vi "State.vi"(7 "State":T1, 8 "error in (no error)":errorcluster, 10 "Data in":variant, 11 "StateData in":T2) -> (0 "error out":errorcluster, 3 "StateData out":T2)   [LabVIEW 2019, in "Project Properties.lvlib"]
doc: "Handles the <b>State</b> command.\n\nCreated by: Ryan Pacini"
uses:
  Project Properties.lvlib
  State Data.ctl
  VI Property.ctl
  State.ctl
  <vilib>/Utility/miscctls.llb/LVPoint32TypeDef.ctl
  <vilib>/Utility/sysdir.llb/System Directory Type.ctl
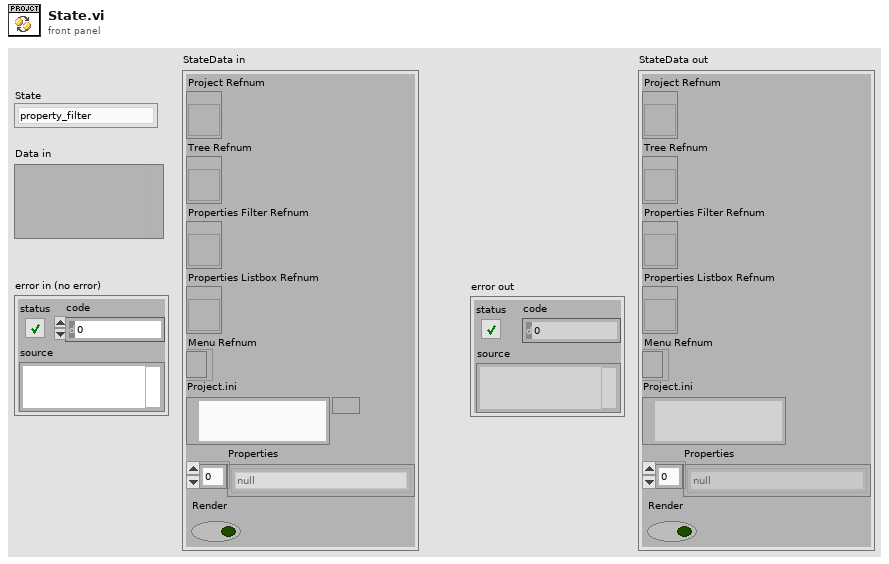
[diagram p1: front panel]
types:
  T1 = typedef "Project Properties.lvlib/State.ctl" = enum8{"property_filter", "property_select", "property_menu_activation", "property_menu_selection", "tree_double_click", "tree_menu_activation", "tree_menu_selection", "export_config"}
  T2 = typedef "Project Properties.lvlib/State Data.ctl" = cluster{"Project Refnum":refnum<vi>, "Tree Refnum":refnum<vi>, "Properties Filter Refnum":refnum<vi>, "Properties Listbox Refnum":refnum<vi>, "Menu Refnum":refnum<k9>, "Project.ini":path, "Properties":T3[], "Render":bool}
  T3 = typedef "Project Properties.lvlib/VI Property.ctl" = enum8{"null", "Auto Logging:Log at Finish", "Auto Logging:Log File Path", "Auto Logging:Print at Finish", "Auto Preallocate Arrays and Strings", "Automatic Error Handling", "BD Master Wizard", "Block Diagram", "Block Diagram Window:Alignment Grid Size", "Block Diagram Window:Native Window", "Block Diagram Window:Open", "Block Diagram Window:Origin", "Block Diagram Window:State", "Block Diagram Window:Window Bounds", "Block Diagram Window:Window Interface", "Callers' Names", "Callers' Paths", "Compiled:Code Complexity", "Compiled:Last Compiled With", "Compiler:Generated Code Profiling Result", "Compiler:Generated Code Profiling Settings", "Connector Pane:Checksum Ignore Dynamic Dispatch v2", "Connector Pane:Checksum v3", "Connector Pane:DataType", "Connector Pane:Reference", "Connector Pane:Set", "Contains Compiled Code", "Context:Has Edits In Another Context", "Context:Has Edits In This Context", "Context:Is Reserved In Other Context", "Context:Is Reserved In This Context", "Control VI Type", "Did Recompile InThis Version", "Do Not Show Save Changes Dialog", "Edit Mode On Open", "Execution highlighting?", "Execution:Allow Debugging", "Execution:Close After Call", "Execution:Compiled With SSE", "Execution:Did Compiler Or User Approve Inlining", "Execution:Inline Enum", "Execution:Inline Is Allowed", "Execution:Inline SubVI", "Execution:Inline SubVI If Possible", "Execution:Is Reentrant", "Execution:Preferred Exec System", "Execution:Priority", "Execution:Reentrancy Type", "Execution:Retain Wire Values", "Execution:Run When Opened", "Execution:Show Front Panel On Call", "Execution:Show Front Panel On Load", "Execution:Shrink Large Buffer Threshold", "Execution:Shrink Large Buffers", "Execution:SSE Runtime Optimization", "Execution:State", "Execution:Suspend On Call", "Expand When Dropped As SubVI", "Front Panel", "Front Panel RefNum TD", "Front Panel Window:Alignment Grid Size", "Front Panel Window:Allow Runtime PopUp", "Front Panel Window:Behavior", "Front Panel Window:Closeable", "Front Panel Window:Custom Title", "Front Panel Window:Highlight Return Button", "Front Panel Window:Is Floating", "Front Panel Window:Is Frontmost", "Front Panel Window:Keep Window Proportions", "Front Panel Window:Minimizable", "Front Panel Window:Minimum Size", "Front Panel Window:Monitor", "Front Panel Window:Native Window", "Front Panel Window:Panel Bounds", "Front Panel Window:Resizable", "Front Panel Window:Run VI Transparently", "Front Panel Window:Show Menu Bar", "Front Panel Window:State", "Front Panel Window:Title", "Front Panel Window:Title Bar Visible", "Front Panel Window:Transparency", "Front Panel Window:Window Bounds", "Front Panel Window:Window Interface", "Has MathScript Nodes", "Help:Document Path", "Help:Document Tag", "Help:Document Web URL", "Help:Examples Exist", "Help:Use Web URL", "Hide Instance VI Caption On Drop", "History:Always Add Comments At Save", "History:Entire Text", "History:Prompt for Comments At Close", "History:Prompt for Comments At Save", "History:Record Application Comments", "History:Revision Number", "History:Use Defaults", "Inline Callees", "Is Clone VI", "Is Generic", "Is In Packed Library", "Is Instance", "Is Probe", "Is Running Interactively", "Is Skinned", "Is System VI", "Is VI Paused?", "Is XNode VI", "Item ID", "Ladder VI Needs Scripting", "Library", "Library:Private", "Library:Version", "Metrics:Advanced", "Metrics:Block Diagram Loaded", "Metrics:Code Size", "Metrics:Front Panel Loaded", "Metrics:Number of clones", "Metrics:Size of Block Diagram", "Metrics:Size of Front Panel", "Metrics:Total Data Size", "Modifications:Block Diagram Mods Bitset", "Modifications:Front Panel Mods Bitset", "Modifications:User Changes", "Modifications:VI Modifications Bitset", "Modifications:VI Signatures", "Modifications:VI User Code GUID", "No Clone If Instance VI", "Number of Non-Proxy Callers", "Overload Info", "Owning Application", "Printing:Block Diagram Scaling?", "Printing:Front Panel Scaling?", "Printing:Header Content:Date Printed?", "Printing:Header Content:Modify Date?", "Printing:Header Content:Page Number?", "Printing:Header Content:VI Icon?", "Printing:Header Content:VI Name?", "Printing:Header Content:VI Path?", "Printing:Margins", "Printing:Page Headers?", "Printing:Page Orientation", "Purgative", "Run-Time Menu Path", "Saved Version", "Statechart:Is Sub Panel Editable", "Statechart:Supress Parse", "Suppress Data Manager", "Suppress Instance VI Halo", "Suppress Transact Info", "Suppress Type Prop", "Tagged And Not Edited", "Terminal Bounds[]", "Tool Bar:Show Abort Button", "Tool Bar:Show Free Run Button", "Tool Bar:Show Run Button", "Tool Bar:Visible", "Tool Kit Attr", "VI Clone Name", "VI Compile Time", "VI Description", "VI Linker Errors", "VI Name", "VI Path", "VI Type"}
  T4 = typedef "LVPoint32TypeDef.ctl" = cluster{"Horizontal":i32, "Vertical":i32}
  T5 = enum16{"open", "replace", "create", "open or create", "replace or create", "replace or create with confirmation"}
  T6 = typedef "System Directory Type.ctl" = i32
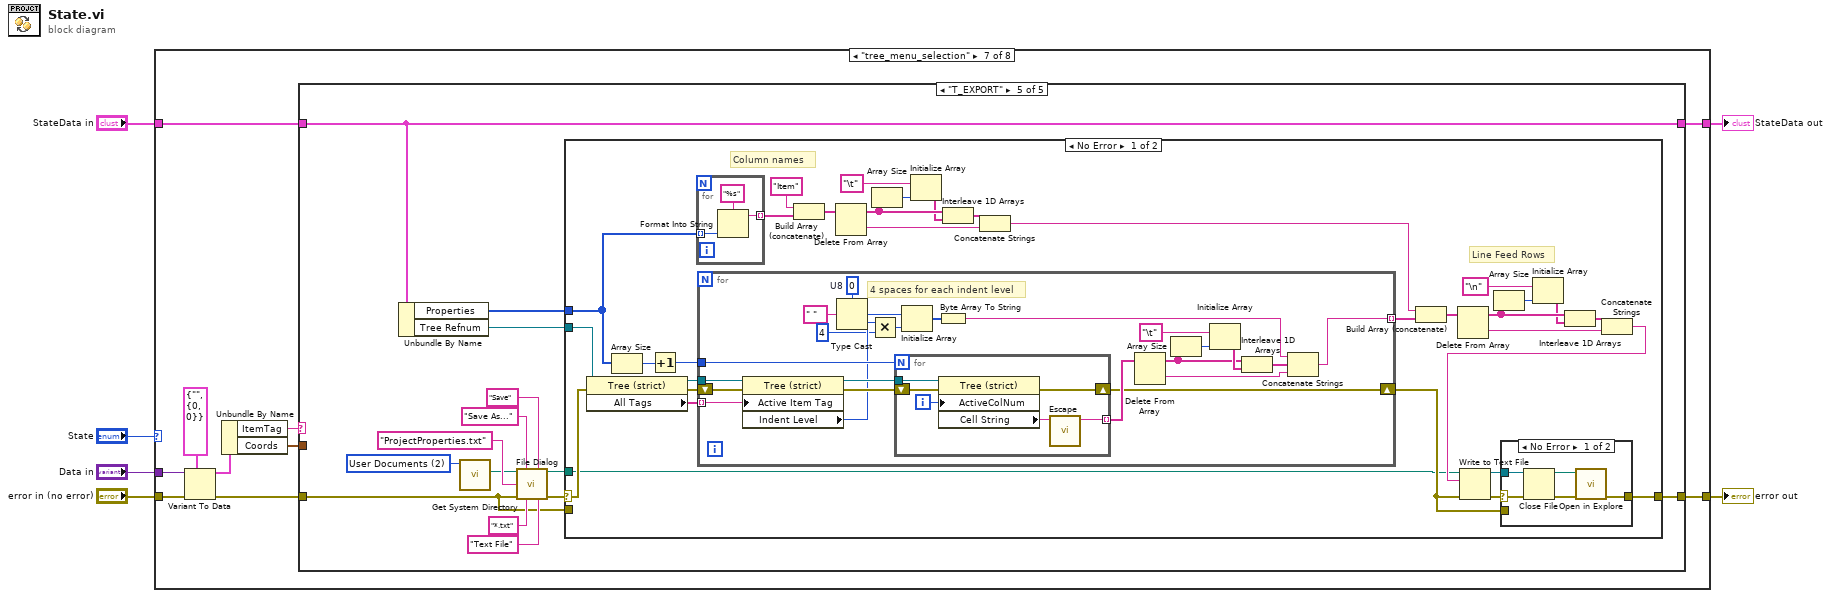
[diagram p0: block diagram]
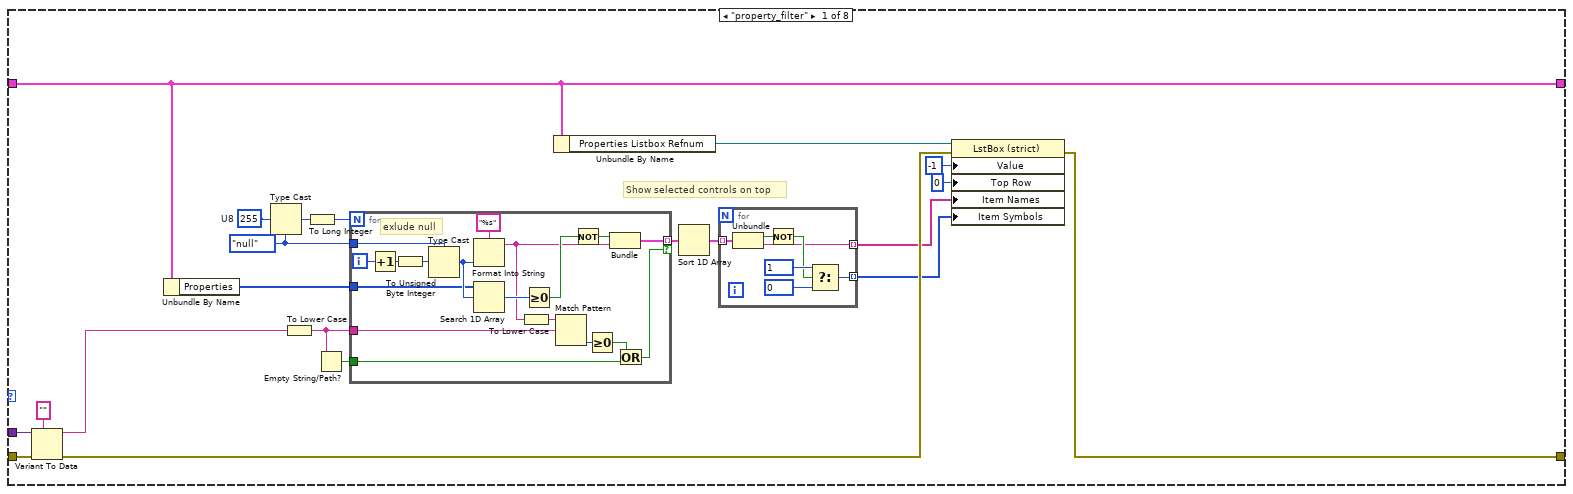
[diagram p2: hidden frame]
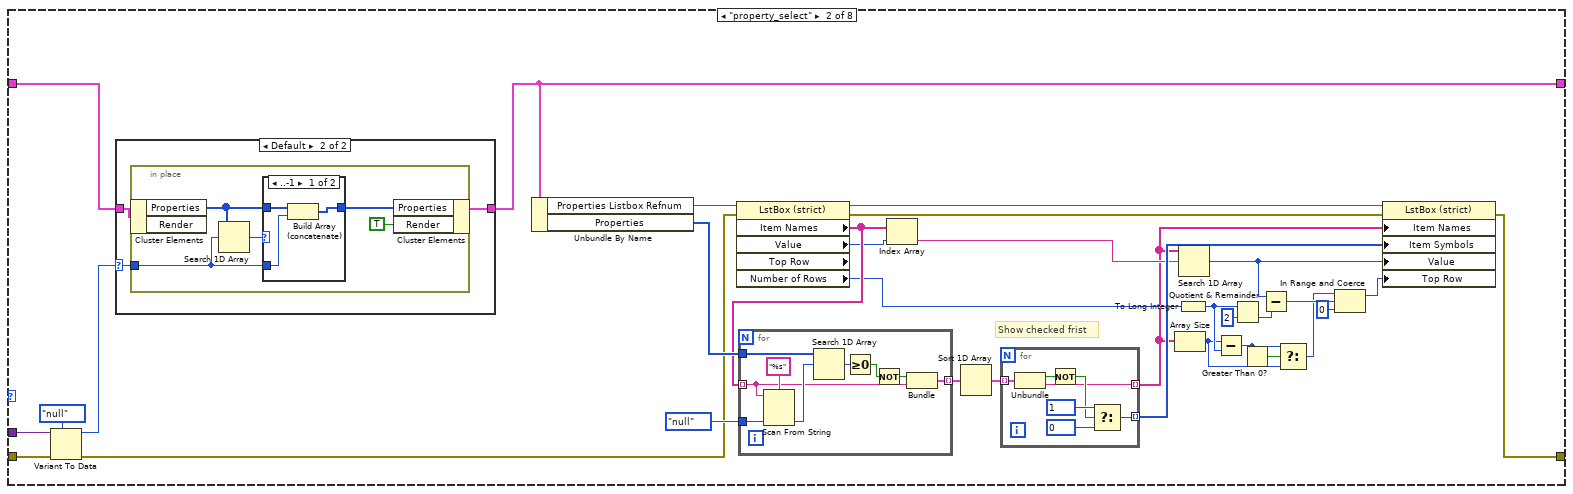
[diagram p3: hidden frame]
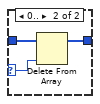
[diagram p5: hidden frame]
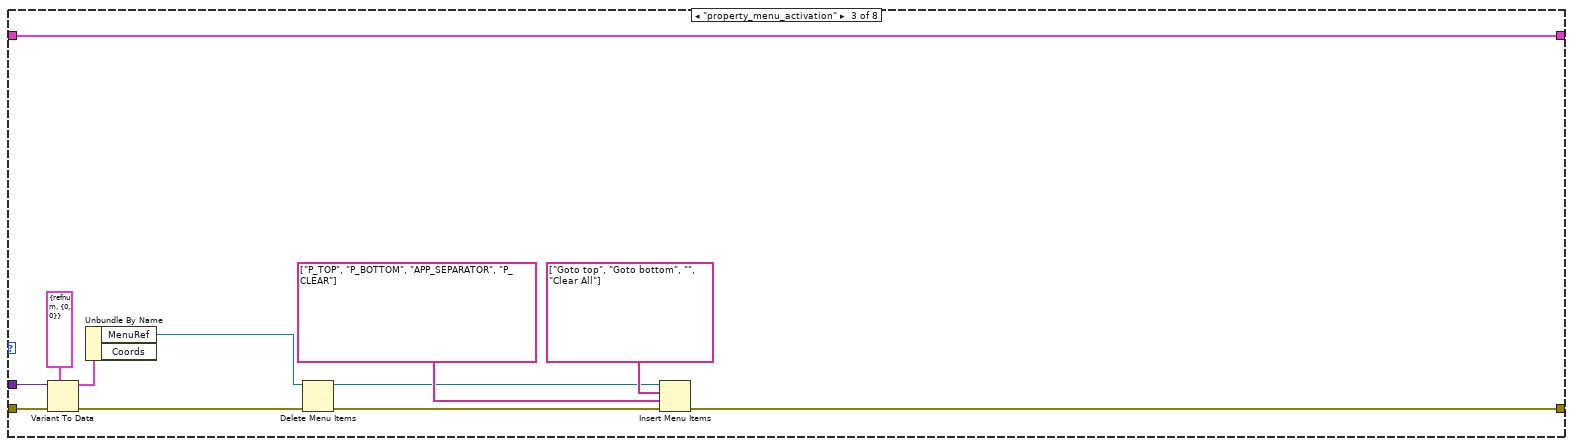
[diagram p6: hidden frame]
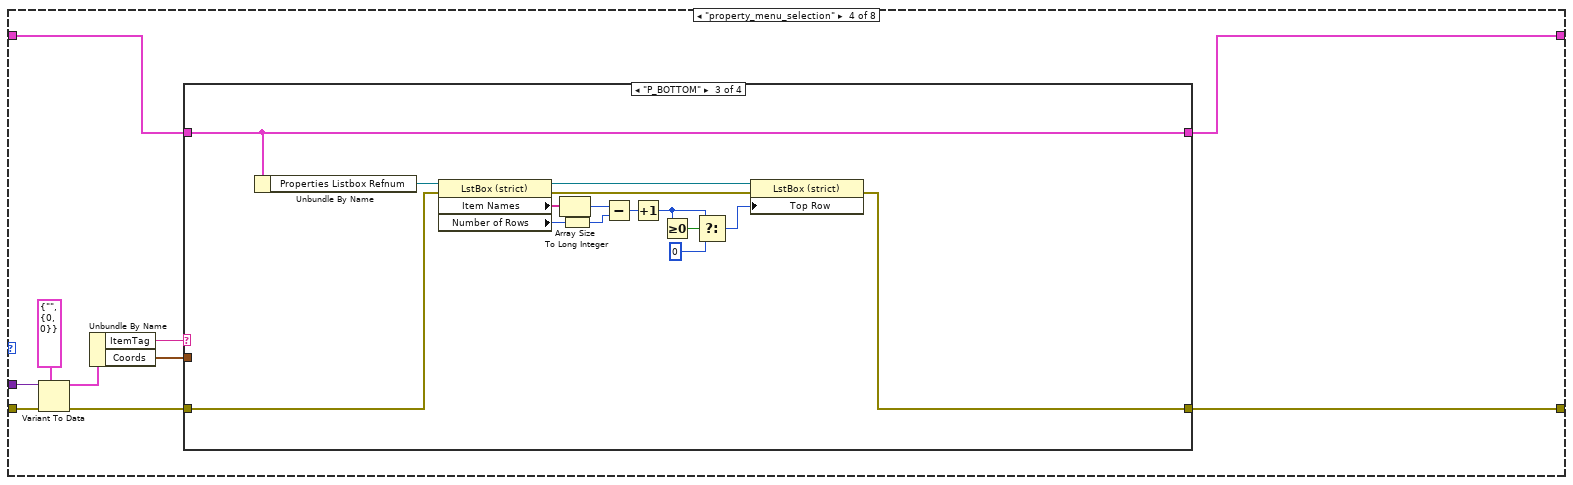
[diagram p7: hidden frame]
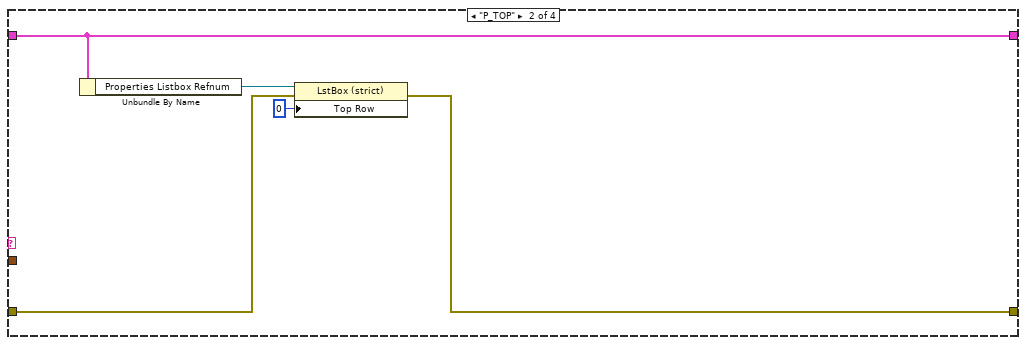
[diagram p9: hidden frame]
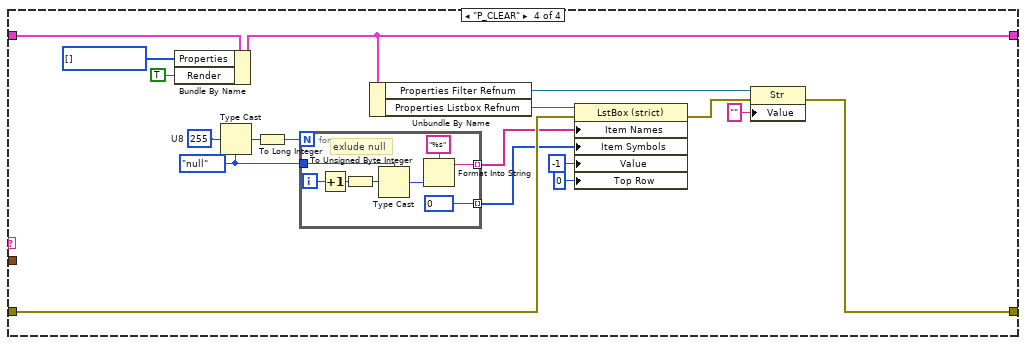
[diagram p10: hidden frame]
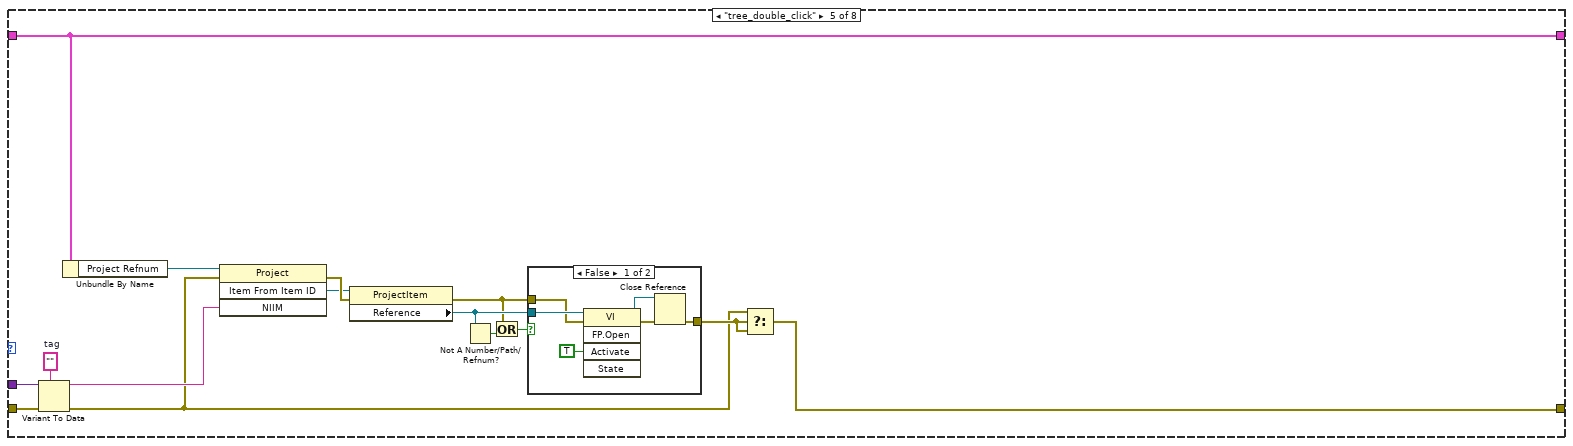
[diagram p11: hidden frame]
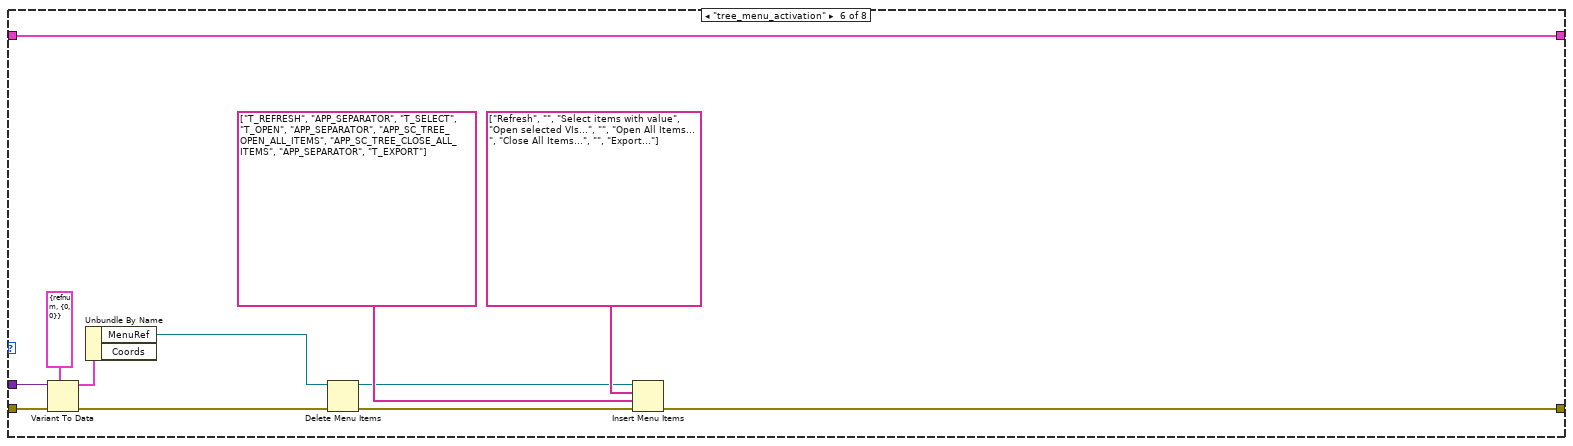
[diagram p13: hidden frame]
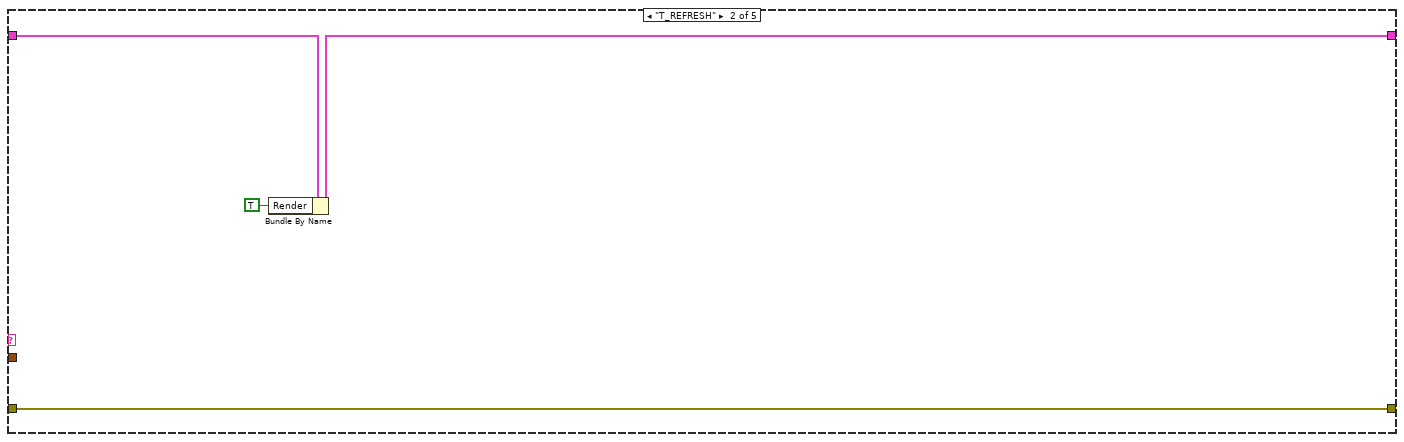
[diagram p15: hidden frame]
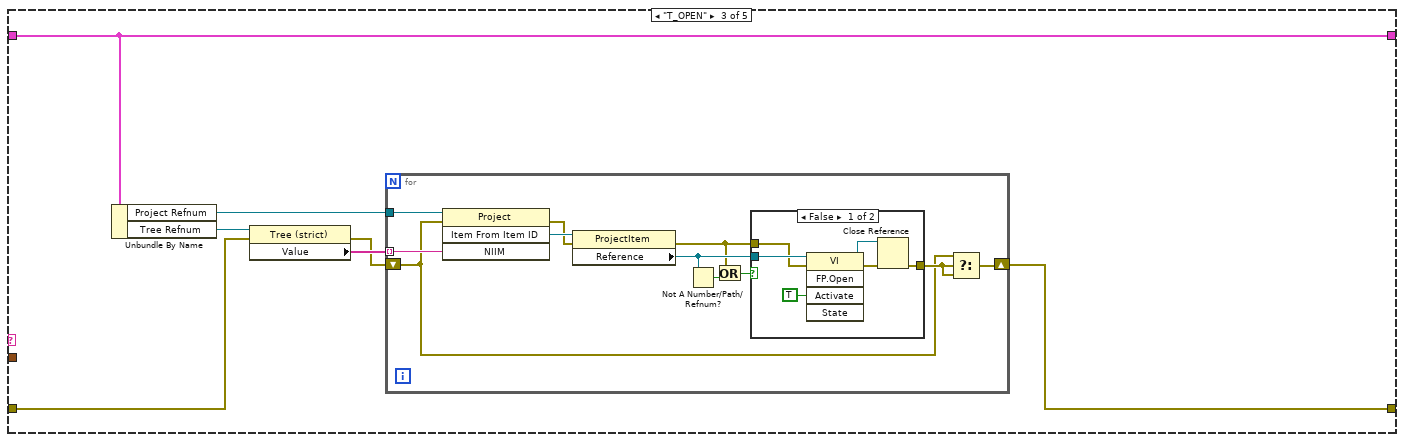
[diagram p16: hidden frame]
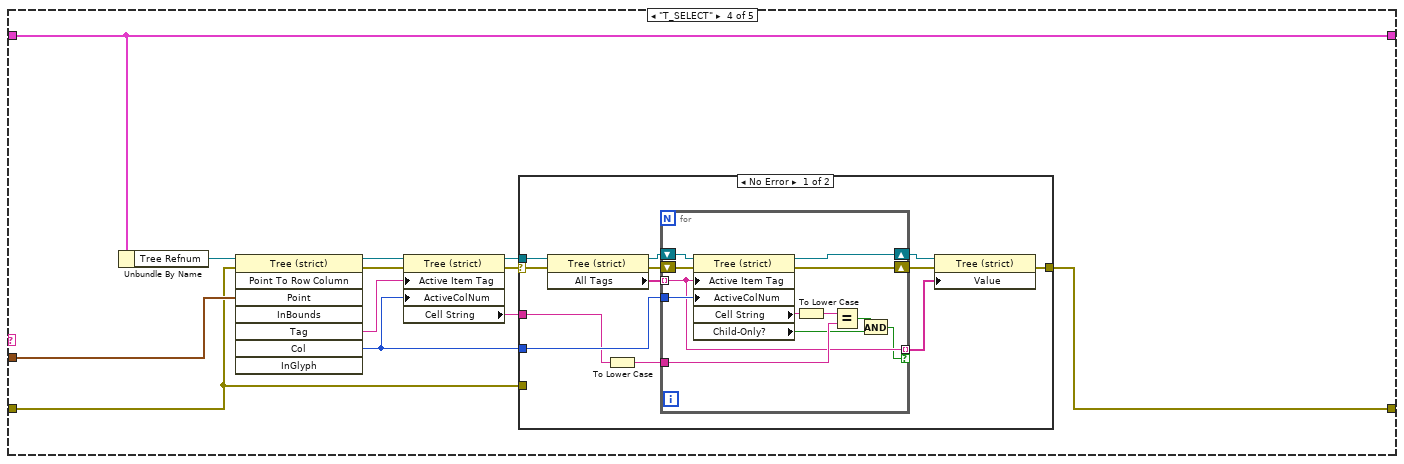
[diagram p18: hidden frame]
diagram:
  n1 = case shown="\"tree_menu_selection\"" "State" {
    tunnel: [w22 w72 w121 w133 w198 w213 w225 w384] -> w6
    tunnel: "error in (no error)" -> [w27 w84 w127 w137 w200 w219 w229 w383]
    tunnel: [w21 w79 w126 w130 w197 w218 w222 w387] -> w4
    tunnel: "StateData in" -> [w21 w80 w126 w131 w197 w218 w223 w387]
    tunnel: "Data in" -> [w26 w83 w125 w136 w199 w217 w228 _]
    frame "property_filter" {
      w19 = u8 255  # U8
      w16 = VI_Property."null" ("VI Property")
      # "Show selected controls on top"
      n2 = Variant To Data(error in=w27, type="", Variant=w26) -> (data=w24:string, error out=w23:errorcluster)
      n3 = Unbundle By Name(w21) -> ("Properties"=w13:T3[])
      n4 = Type Cast(type=w16, x=w19) -> (*(type *) &x=w18:T3)
      n5 = To Lower Case(string=w24) -> (all lower case string=w12:string)
      n6 = To Long Integer(number=w18) -> (32bit integer=w17:i32)
      n7 = Empty String/Path?(string/path=w12) -> (empty?=w11:bool)
      n8 = for {
        N: w17 -> [_]
        tunnel: w16 -> [w49]
        tunnel: [w36] -> w15 mode=indexing if=w39
        tunnel: w13 -> [w42]
        tunnel: w12 -> [w43]
        tunnel: w11 -> [w41]
        i -> [w52]
        # "exlude null"
        n9 = Increment(x=w52) -> (x+1=w51:i32)
        n10 = To Unsigned Byte Integer(number=w51) -> (unsigned 8bit integer=w50:u8)
        n11 = Type Cast(type=w49, x=w50) -> (*(type *) &x=w47:T3)
        n12 = Format Into String(format string="%s", w47) -> (resulting string=w37:string)  [unwired: 2 in, 1 out]
        n13 = Search 1D Array(1D array=w42, element=w47) -> (index of element=w46:i32)  [unwired: 1 in]
        n14 = To Lower Case(string=w37) -> (all lower case string=w45:string)
        n15 = Greater Or Equal To 0?(x=w46) -> (x >= 0?=w38:bool)
        n16 = Match Pattern(string=w45, regular expression=w43) -> (offset past match=w44:i32)  [unwired: 1 in, 3 out]
        n17 = Not(x=w38) -> (.not. x?=w35:bool)
        n18 = Greater Or Equal To 0?(x=w44) -> (x >= 0?=w40:bool)
        n19 = Bundle(w35, w37) -> (w36:cluster{bool, string})  [unwired: 1 in]
        n20 = Or(x=w40, y=w41) -> (x .or. y?=w39:bool)
      }
      n21 = Unbundle By Name(w21) -> ("Properties Listbox Refnum"=w20:refnum<vi>)
      n22 = Sort 1D Array(array=w15) -> (sorted array=w9:cluster{bool, string}[])
      n23 = for {
        tunnel: w9 -> [w34] mode=indexing
        tunnel: [w29] -> w8 mode=indexing
        tunnel: [w28] -> w7 mode=indexing
        n24 = Unbundle(w34) -> (w33:bool, w29:string)
        n25 = Not(x=w33) -> (.not. x?=w30:bool)
        n26 = Select(t=1, s=w30, f=0) -> (s? t:f=w28:i32)
      }
      n27 = property class="LstBox (strict)"(reference=w20, error in=w23, "Value"=-1, "Top Row"=0, "Item Names"=w8, "Item Symbols"=w7) -> (error out=w22:errorcluster)  [unwired: 1 out]
    }
    frame "property_select" {
      # "Show checked frist"
      n28 = Variant To Data(error in=w84, type=VI_Property."null" ("VI Property"), Variant=w83) -> (data=w81:T3, error out=w73:errorcluster)
      n29 = case shown="Default" w81 {
        selector: w81 -> [_ w103]
        tunnel: w80 -> [w101 w104]
        tunnel: [w101 w102] -> w79
        frame "null" {
        }
        frame Default {
          n30 = in-place {
            in-place-border: w103 -> [w106]
            n31 = in-place-cluster #1(w104) -> ("Properties"=w108:T3[])  [unwired: 1 out]
            n32 = Search 1D Array(1D array=w108, element=w106) -> (index of element=w109:i32)  [unwired: 1 in]
            n33 = case shown="..-1" w109 {
              selector: w109 -> [_ w114]
              tunnel: w108 -> [w112 w115]
              tunnel: [w111 w113] -> w107
              tunnel: w106 -> [w110 _]
              frame ..-1 {
                n34 = Build Array (concatenate)(w112, w110) -> (w111:T3[])
              }
              frame 0.. {
                n35 = Delete From Array(array=w115, index=w114) -> (array with subset deleted=w113:T3[])  [unwired: 1 in, 1 out]
              }
            }
            n36 = in-place-cluster #1("Properties"=w107, "Render"=TRUE) -> (w102:T2)
          }
        }
      }
      n37 = Unbundle By Name(w79) -> ("Properties Listbox Refnum"=w78:refnum<vi>, "Properties"=w76:T3[])
      n38 = property class="LstBox (strict)" props=["Item Names", "Value", "Top Row", "Number of Rows"](reference=w78, error in=w73) -> (reference out=w74:refnum<vi>, error out=w75:errorcluster, "Item Names"=w68:string[], "Value"=w66:i32, "Number of Rows"=w64:u32)  [unwired: 1 out]
      n39 = for {
        tunnel: w68 -> [w94] mode=indexing
        tunnel: VI_Property."null" ("VI Property") -> [w100]
        tunnel: w76 -> [w97]
        tunnel: [w93] -> w70 mode=indexing
        n40 = Scan From String(format string="%s", input string=w94, default 1=w100) -> (output 1=w98:T3)  [unwired: 2 in, 3 out]
        n41 = Search 1D Array(1D array=w97, element=w98) -> (index of element=w96:i32)  [unwired: 1 in]
        n42 = Greater Or Equal To 0?(x=w96) -> (x >= 0?=w95:bool)
        n43 = Not(x=w95) -> (.not. x?=w92:bool)
        n44 = Bundle(w92, w94) -> (w93:cluster{bool, string})  [unwired: 1 in]
      }
      n45 = Index Array(array=w68, index=w66) -> (element=w67:string)
      n46 = Sort 1D Array(array=w70) -> (sorted array=w71:cluster{bool, string}[])
      n47 = for {
        tunnel: w71 -> [w91] mode=indexing
        tunnel: [w86] -> w61 mode=indexing
        tunnel: [w85] -> w69 mode=indexing
        n48 = Unbundle(w91) -> (w90:bool, w86:string)
        n49 = Not(x=w90) -> (.not. x?=w87:bool)
        n50 = Select(t=1, s=w87, f=0) -> (s? t:f=w85:i32)
      }
      n51 = Array Size(array=w61) -> (size(s)=w53:i32)
      n52 = To Long Integer(number=w64) -> (32bit integer=w59:i32)
      n53 = Search 1D Array(1D array=w61, element=w67) -> (index of element=w65:i32)  [unwired: 1 in]
      n54 = Subtract(x=w53, y=w59) -> (x-y=w55:i32)
      n55 = Quotient & Remainder(x=w59, y=2) -> (floor(x/y)=w58:i32)  [unwired: 1 out]
      n56 = Greater Than 0?(x=w55) -> (x > 0?=w56:bool)
      n57 = Subtract(x=w65, y=w58) -> (x-y=w63:i32)
      n58 = Select(t=w55, s=w56, f=w53) -> (s? t:f=w54:i32)
      n59 = In Range and Coerce(upper limit=w54, x=w63, lower limit=0) -> (coerced(x)=w60:i32)  [unwired: 1 out]
      n60 = property class="LstBox (strict)"(reference=w74, error in=w75, "Item Names"=w61, "Item Symbols"=w69, "Value"=w65, "Top Row"=w60) -> (error out=w72:errorcluster)  [unwired: 1 out]
    }
    frame "property_menu_activation" {
      n61 = Variant To Data(error in=w127, type=cluster{"MenuRef":refnum<k9>, "Coords":T4} {"MenuRef"=refnum, "Coords"={"Horizontal"=0, "Vertical"=0}} ("output cluster"), Variant=w125) -> (data=w123:cluster{"MenuRef":refnum<k9>, "Coords":T4}, error out=w122:errorcluster)
      n62 = Unbundle By Name(w123) -> ("MenuRef"=w117:refnum<k9>)  [unwired: 1 out]
      n63 = Delete Menu Items(6:w122, 9:w117) -> (0:w118:errorcluster, 3:w116:refnum<k9>)  [unwired: 2 in]
      n64 = Insert Menu Items(6:w118, 7:string[] ["P_TOP", "P_BOTTOM", "APP_SEPARATOR", "P_CLEAR"], 8:string[] ["Goto top", "Goto bottom", "", "Clear All"], 9:w116) -> (0:w121:errorcluster)  [unwired: 2 in, 2 out]
    }
    frame "property_menu_selection" {
      n65 = Variant To Data(error in=w137, type=cluster{"ItemTag":string, "Coords":T4} {"ItemTag"="", "Coords"={"Horizontal"=0, "Vertical"=0}} ("output cluster"), Variant=w136) -> (data=w134:cluster{"ItemTag":string, "Coords":T4}, error out=w132:errorcluster)
      n66 = Unbundle By Name(w134) -> ("ItemTag"=w129:string, "Coords"=w128:T4)
      n67 = case shown="\"P_BOTTOM\"" w129 {
        tunnel: [w138 w142 w157 w162] -> w133
        tunnel: w132 -> [w138 w141 w147 w172]
        tunnel: [w139 w144 w159 w175] -> w130
        tunnel: w131 -> [w139 w144 w159 w177]
        tunnel: w128 -> [_ _ _ _]
        frame Default {
        }
        frame "P_TOP" {
          n68 = Unbundle By Name(w144) -> ("Properties Listbox Refnum"=w143:refnum<vi>)
          n69 = property class="LstBox (strict)"(reference=w143, error in=w141, "Top Row"=0) -> (error out=w142:errorcluster)  [unwired: 1 out]
        }
        frame "P_BOTTOM" {
          n70 = Unbundle By Name(w159) -> ("Properties Listbox Refnum"=w158:refnum<vi>)
          n71 = property class="LstBox (strict)"(reference=w158, error in=w147) -> (reference out=w156:refnum<vi>, error out=w146:errorcluster, "Item Names"=w155:string[], "Number of Rows"=w153:u32)
          n72 = Array Size(array=w155) -> (size(s)=w154:i32)
          n73 = To Long Integer(number=w153) -> (32bit integer=w152:i32)
          n74 = Subtract(x=w154, y=w152) -> (x-y=w150:i32)
          n75 = Increment(x=w150) -> (x+1=w145:i32)
          n76 = Greater Or Equal To 0?(x=w145) -> (x >= 0?=w151:bool)
          n77 = Select(t=w145, s=w151, f=0) -> (s? t:f=w148:i32)
          n78 = property class="LstBox (strict)"(reference=w156, error in=w146, "Top Row"=w148) -> (error out=w157:errorcluster)  [unwired: 1 out]
        }
        frame "P_CLEAR" {
          w170 = u8 255  # U8
          w167 = VI_Property."null" ("VI Property")
          w174 = T3[] [] items=["null", "Auto Logging:Log at Finish", "Auto Logging:Log File Path", "Auto Logging:Print at Finish", "Auto Preallocate Arrays and Strings", "Automatic Error Handling", "BD Master Wizard", "Block Diagram", "Block Diagram Window:Alignment Grid Size", "Block Diagram Window:Native Window", "Block Diagram Window:Open", "Block Diagram Window:Origin", "Block Diagram Window:State", "Block Diagram Window:Window Bounds", "Block Diagram Window:Window Interface", "Callers' Names", "Callers' Paths", "Compiled:Code Complexity", "Compiled:Last Compiled With", "Compiler:Generated Code Profiling Result", "Compiler:Generated Code Profiling Settings", "Connector Pane:Checksum Ignore Dynamic Dispatch v2", "Connector Pane:Checksum v3", "Connector Pane:DataType", "Connector Pane:Reference", "Connector Pane:Set", "Contains Compiled Code", "Context:Has Edits In Another Context", "Context:Has Edits In This Context", "Context:Is Reserved In Other Context", "Context:Is Reserved In This Context", "Control VI Type", "Did Recompile InThis Version", "Do Not Show Save Changes Dialog", "Edit Mode On Open", "Execution highlighting?", "Execution:Allow Debugging", "Execution:Close After Call", "Execution:Compiled With SSE", "Execution:Did Compiler Or User Approve Inlining", "Execution:Inline Enum", "Execution:Inline Is Allowed", "Execution:Inline SubVI", "Execution:Inline SubVI If Possible", "Execution:Is Reentrant", "Execution:Preferred Exec System", "Execution:Priority", "Execution:Reentrancy Type", "Execution:Retain Wire Values", "Execution:Run When Opened", "Execution:Show Front Panel On Call", "Execution:Show Front Panel On Load", "Execution:Shrink Large Buffer Threshold", "Execution:Shrink Large Buffers", "Execution:SSE Runtime Optimization", "Execution:State", "Execution:Suspend On Call", "Expand When Dropped As SubVI", "Front Panel", "Front Panel RefNum TD", "Front Panel Window:Alignment Grid Size", "Front Panel Window:Allow Runtime PopUp", "Front Panel Window:Behavior", "Front Panel Window:Closeable", "Front Panel Window:Custom Title", "Front Panel Window:Highlight Return Button", "Front Panel Window:Is Floating", "Front Panel Window:Is Frontmost", "Front Panel Window:Keep Window Proportions", "Front Panel Window:Minimizable", "Front Panel Window:Minimum Size", "Front Panel Window:Monitor", "Front Panel Window:Native Window", "Front Panel Window:Panel Bounds", "Front Panel Window:Resizable", "Front Panel Window:Run VI Transparently", "Front Panel Window:Show Menu Bar", "Front Panel Window:State", "Front Panel Window:Title", "Front Panel Window:Title Bar Visible", "Front Panel Window:Transparency", "Front Panel Window:Window Bounds", "Front Panel Window:Window Interface", "Has MathScript Nodes", "Help:Document Path", "Help:Document Tag", "Help:Document Web URL", "Help:Examples Exist", "Help:Use Web URL", "Hide Instance VI Caption On Drop", "History:Always Add Comments At Save", "History:Entire Text", "History:Prompt for Comments At Close", "History:Prompt for Comments At Save", "History:Record Application Comments", "History:Revision Number", "History:Use Defaults", "Inline Callees", "Is Clone VI", "Is Generic", "Is In Packed Library", "Is Instance", "Is Probe", "Is Running Interactively", "Is Skinned", "Is System VI", "Is VI Paused?", "Is XNode VI", "Item ID", "Ladder VI Needs Scripting", "Library", "Library:Private", "Library:Version", "Metrics:Advanced", "Metrics:Block Diagram Loaded", "Metrics:Code Size", "Metrics:Front Panel Loaded", "Metrics:Number of clones", "Metrics:Size of Block Diagram", "Metrics:Size of Front Panel", "Metrics:Total Data Size", "Modifications:Block Diagram Mods Bitset", "Modifications:Front Panel Mods Bitset", "Modifications:User Changes", "Modifications:VI Modifications Bitset", "Modifications:VI Signatures", "Modifications:VI User Code GUID", "No Clone If Instance VI", "Number of Non-Proxy Callers", "Overload Info", "Owning Application", "Printing:Block Diagram Scaling?", "Printing:Front Panel Scaling?", "Printing:Header Content:Date Printed?", "Printing:Header Content:Modify Date?", "Printing:Header Content:Page Number?", "Printing:Header Content:VI Icon?", "Printing:Header Content:VI Name?", "Printing:Header Content:VI Path?", "Printing:Margins", "Printing:Page Headers?", "Printing:Page Orientation", "Purgative", "Run-Time Menu Path", "Saved Version", "Statechart:Is Sub Panel Editable", "Statechart:Supress Parse", "Suppress Data Manager", "Suppress Instance VI Halo", "Suppress Transact Info", "Suppress Type Prop", "Tagged And Not Edited", "Terminal Bounds[]", "Tool Bar:Show Abort Button", "Tool Bar:Show Free Run Button", "Tool Bar:Show Run Button", "Tool Bar:Visible", "Tool Kit Attr", "VI Clone Name", "VI Compile Time", "VI Description", "VI Linker Errors", "VI Name", "VI Path", "VI Type"] ("Properties")
          n79 = Bundle By Name(cluster=w177, "Properties"=w174, "Render"=TRUE) -> (w175:T2)
          n80 = Type Cast(type=w167, x=w170) -> (*(type *) &x=w169:T3)
          n81 = To Long Integer(number=w169) -> (32bit integer=w168:i32)
          n82 = for {
            N: w168 -> [_]
            tunnel: w167 -> [w182]
            tunnel: [w179] -> w166 mode=indexing
            tunnel: [0] -> w165 mode=indexing
            i -> [w185]
            # "exlude null"
            n83 = Increment(x=w185) -> (x+1=w184:i32)
            n84 = To Unsigned Byte Integer(number=w184) -> (unsigned 8bit integer=w183:u8)
            n85 = Type Cast(type=w182, x=w183) -> (*(type *) &x=w180:T3)
            n86 = Format Into String(format string="%s", w180) -> (resulting string=w179:string)  [unwired: 2 in, 1 out]
          }
          n87 = Unbundle By Name(w175) -> ("Properties Filter Refnum"=w161:refnum<vi>, "Properties Listbox Refnum"=w176:refnum<vi>)
          n88 = property class="LstBox (strict)"(reference=w176, error in=w172, "Item Names"=w166, "Item Symbols"=w165, "Value"=-1, "Top Row"=0) -> (error out=w171:errorcluster)  [unwired: 1 out]
          n89 = property class="Str"(reference=w161, error in=w171, "Value"="") -> (error out=w162:errorcluster)  [unwired: 1 out]
        }
      }
    }
    frame "tree_double_click" {
      w189 = ""  # tag
      n90 = Variant To Data(error in=w200, type=w189, Variant=w199) -> (data=w188:string, error out=w187:errorcluster)
      n91 = Unbundle By Name(w197) -> ("Project Refnum"=w196:refnum<vi>)
      n92 = invoke class="Project" method="Item From Item ID"(reference=w196, error in=w187, "NIIM"=w188) -> (error out=w195:errorcluster, "GetItemFromNIIM"=w186:refnum<vi>)  [unwired: 1 in, 2 out]
      n93 = property class="ProjectItem"(reference=w186, error in=w195) -> (error out=w192:errorcluster, "Reference"=w193:refnum<vi>)  [unwired: 1 out]
      n94 = Not A Number/Path/Refnum?(number/path/refnum=w193) -> (NaN/Path/Refnum?=w194:bool)
      n95 = Or(x=w192, y=w194) -> (x .or. y?=w191:bool)
      n96 = case shown="False" w191 {
        tunnel: w193 -> [w206 _]
        tunnel: w192 -> [w204 w207]
        tunnel: [w201 w207] -> w190
        frame False {
          n97 = invoke class="VI" method="FP.Open"(reference=w206, error in=w204, "Activate"=TRUE ("Activate?")) -> (reference out=w202:refnum<vi>, error out=w203:errorcluster)  [unwired: 2 in, 3 out]
          n98 = Close Reference(reference=w202, error in (no error)=w203) -> (error out=w201:errorcluster)
        }
        frame True {
        }
      }
      n99 = Select(t=w187, s=w190, f=w190) -> (s? t:f=w198:errorcluster)
    }
    frame "tree_menu_activation" {
      n100 = Variant To Data(error in=w219, type=cluster{"MenuRef":refnum<k9>, "Coords":T4} {"MenuRef"=refnum, "Coords"={"Horizontal"=0, "Vertical"=0}} ("output cluster"), Variant=w217) -> (data=w215:cluster{"MenuRef":refnum<k9>, "Coords":T4}, error out=w214:errorcluster)
      n101 = Unbundle By Name(w215) -> ("MenuRef"=w209:refnum<k9>)  [unwired: 1 out]
      n102 = Delete Menu Items(6:w214, 9:w209) -> (0:w210:errorcluster, 3:w208:refnum<k9>)  [unwired: 2 in]
      n103 = Insert Menu Items(6:w210, 7:string[] ["T_REFRESH", "APP_SEPARATOR", "T_SELECT", "T_OPEN", "APP_SEPARATOR", "APP_SC_TREE_OPEN_ALL_ITEMS", "APP_SC_TREE_CLOSE_ALL_ITEMS", "APP_SEPARATOR", "T_EXPORT"], 8:string[] ["Refresh", "", "Select items with value", "Open selected VIs...", "", "Open All Items...", "Close All Items...", "", "Export..."], 9:w208) -> (0:w213:errorcluster)  [unwired: 2 in, 2 out]
    }
    frame "tree_menu_selection" {
      n104 = Variant To Data(error in=w229, type=cluster{"ItemTag":string, "Coords":T4} {"ItemTag"="", "Coords"={"Horizontal"=0, "Vertical"=0}} ("output cluster"), Variant=w228) -> (data=w226:cluster{"ItemTag":string, "Coords":T4}, error out=w224:errorcluster)
      n105 = Unbundle By Name(w226) -> ("ItemTag"=w221:string, "Coords"=w220:T4)
      n106 = case shown="\"T_EXPORT\"" w221 {
        tunnel: [w230 w235 w240 w262 w308] -> w225
        tunnel: w224 -> [w230 w235 w236 w261 w298]
        tunnel: [w231 w233 w242 w270 w311] -> w222
        tunnel: w223 -> [w231 w234 w242 w270 w311]
        tunnel: w220 -> [_ _ _ w271 _]
        frame Default {
        }
        frame "T_REFRESH" {
          n107 = Bundle By Name(cluster=w234, "Render"=TRUE) -> (w233:T2)
        }
        frame "T_OPEN" {
          n108 = Unbundle By Name(w242) -> ("Project Refnum"=w241:refnum<vi>, "Tree Refnum"=w239:refnum<vi>)
          n109 = property class="Tree (strict)"(reference=w239, error in=w236) -> (error out=w237:errorcluster, "Value"=w238:string[])  [unwired: 1 out]
          n110 = for {
            tunnel: w241 -> [w253]
            tunnel: w238 -> [w244] mode=indexing
            shift-right: [w245] -> w240
            shift-left: w237 -> [w243]
            n111 = invoke class="Project" method="Item From Item ID"(reference=w253, error in=w243, "NIIM"=w244) -> (error out=w251:errorcluster, "GetItemFromNIIM"=w252:refnum<vi>)  [unwired: 1 in, 2 out]
            n112 = property class="ProjectItem"(reference=w252, error in=w251) -> (error out=w248:errorcluster, "Reference"=w249:refnum<vi>)  [unwired: 1 out]
            n113 = Not A Number/Path/Refnum?(number/path/refnum=w249) -> (NaN/Path/Refnum?=w250:bool)
            n114 = Or(x=w248, y=w250) -> (x .or. y?=w247:bool)
            n115 = case shown="False" w247 {
              tunnel: w249 -> [w259 _]
              tunnel: w248 -> [w257 w260]
              tunnel: [w254 w260] -> w246
              frame False {
                n116 = invoke class="VI" method="FP.Open"(reference=w259, error in=w257, "Activate"=TRUE ("Activate?")) -> (reference out=w255:refnum<vi>, error out=w256:errorcluster)  [unwired: 2 in, 3 out]
                n117 = Close Reference(reference=w255, error in (no error)=w256) -> (error out=w254:errorcluster)
              }
              frame True {
              }
            }
            n118 = Select(t=w243, s=w246, f=w246) -> (s? t:f=w245:errorcluster)
          }
        }
        frame "T_SELECT" {
          n119 = Unbundle By Name(w270) -> ("Tree Refnum"=w272:refnum<vi>)
          n120 = invoke class="Tree (strict)" method="Point To Row Column"(reference=w272, error in=w261, "Point"=w271) -> (reference out=w269:refnum<vi>, error out=w267:errorcluster, "Tag"=w266:string, "Col"=w265:i32)  [unwired: 5 in, 4 out]
          n121 = property class="Tree (strict)"(reference=w269, error in=w267, "Active Item Tag"=w266, "ActiveColNum"=w265) -> (reference out=w268:refnum<vi>, error out=w263:errorcluster, "Cell String"=w264:string)
          n122 = case shown="No Error" w263 {
            selector: w263 -> [w276 _]
            tunnel: w268 -> [w281 _]
            tunnel: w265 -> [w280 _]
            tunnel: w264 -> [w278 _]
            tunnel: [w275 w297] -> w262
            tunnel: w261 -> [_ w297]
            frame No Error {
              n123 = property class="Tree (strict)"(reference=w281, error in=w276) -> (reference out=w284:refnum<vi>, error out=w283:errorcluster, "All Tags"=w282:string[])
              n124 = To Lower Case(string=w278) -> (all lower case string=w277:string)
              n125 = for {
                tunnel: w282 -> [w287] mode=indexing
                tunnel: [w287] -> w273 mode=indexing if=w286
                shift-right: [w294] -> w274
                shift-left: w284 -> [w296]
                shift-right: [w293] -> w279
                shift-left: w283 -> [w295]
                tunnel: w280 -> [w292]
                tunnel: w277 -> [w288]
                n126 = property class="Tree (strict)"(reference=w296, error in=w295, "Active Item Tag"=w287, "ActiveColNum"=w292) -> (reference out=w294:refnum<vi>, error out=w293:errorcluster, "Cell String"=w291:string, "Child-Only?"=w285:bool)
                n127 = To Lower Case(string=w291) -> (all lower case string=w289:string)
                n128 = Equal?(x=w289, y=w288) -> (x = y?=w290:bool)
                n129 = And(x=w290, y=w285) -> (x .and. y?=w286:bool)
              }
              n130 = property class="Tree (strict)"(reference=w274, error in=w279, "Value"=w273) -> (error out=w275:errorcluster)  [unwired: 1 out]
            }
            frame Error {
              # "Do nothing on failure"
            }
          }
        }
        frame "T_EXPORT" {
          w302 = T6 2 items=["User Home"=0, "User Desktop"=1, "User Documents"=2, "User Application Data"=3, "User Preferences"=4, "User Temporary"=5, "Public Documents"=6, "Public Application Data"=7, "Public Preferences"=8, "Public Cache"=13, "System Core Libraries"=9, "System Installed Libraries"=10, "Application Files"=11, "Boot Volume Root"=12] ("system directory type")
          n131 = Unbundle By Name(w311) -> ("Properties"=w309:T3[], "Tree Refnum"=w310:refnum<vi>)
          n132 = call <vilib>:"Get System Directory.vi"("system directory type"=w302) -> ("system directory"=w301:path)  [unwired: 10 in]
          n133 = call "File Dialog"("start path"=w301, "prompt"="Save As...", "button label"="Save", "default name"="ProjectProperties.txt", "error in"=w298, "pattern (all files)"="*.txt", "pattern label"="Text File") -> ("selected path"=w299:path, "error out"=w300:errorcluster)  [unwired: 5 in, 2 out]
          n134 = case shown="No Error" w300 {
            selector: w300 -> [w318 _]
            tunnel: w310 -> [w343 _]
            tunnel: w309 -> [w337 _]
            tunnel: w298 -> [_ w382]
            tunnel: w299 -> [w312 _]
            tunnel: [w314 w382] -> w308
            frame No Error {
              # "Line Feed Rows"
              # "Column names"
              n135 = property class="Tree (strict)"(reference=w343, error in=w318) -> (reference out=w342:refnum<vi>, error out=w341:errorcluster, "All Tags"=w340:string[])
              n136 = Array Size(array=w337) -> (size(s)=w339:i32)
              n137 = Increment(x=w339) -> (x+1=w338:i32)
              n138 = for {
                tunnel: w337 -> [w352] mode=indexing
                tunnel: [w350] -> w336 mode=indexing
                n139 = Format Into String(format string="%s", w352) -> (resulting string=w350:string)  [unwired: 2 in, 1 out]
              }
              n140 = for {
                tunnel: w342 -> [w375]
                tunnel: w340 -> [w373] mode=indexing
                tunnel: w338 -> [w372]
                shift-right: [w362] -> w313
                shift-left: w341 -> [w374]
                tunnel: [w361] -> w321 mode=indexing
                w357 = u8 0  # U8
                # "4 spaces for each indent level"
                n141 = property class="Tree (strict)"(reference=w375, error in=w374, "Active Item Tag"=w373) -> (reference out=w365:refnum<vi>, error out=w364:errorcluster, "Indent Level"=w360:i32)
                n142 = Type Cast(type=w357, x=" ") -> (*(type *) &x=w358:u8)
                n143 = Multiply(x=w360, y=4 ("x")) -> (x*y=w356:i32)
                n144 = for {
                  N: w372 -> [_]
                  tunnel: w365 -> [w381]
                  tunnel: [w376] -> w363 mode=indexing
                  shift-right: [w378] -> w362
                  shift-left: w364 -> [w380]
                  i -> [w379]
                  n145 = property class="Tree (strict)"(reference=w381, error in=w380, "ActiveColNum"=w379) -> (error out=w378:errorcluster, "Cell String"=w377:string)  [unwired: 1 out]
                  n146 = call "Escape.vi"("string"=w377) -> ("escaped string"=w376:string)  [unwired: 9 in, 1 out]
                }
                n147 = Initialize Array(w358, w356) -> (w354:u8[])
                n148 = Byte Array To String(unsigned byte array=w354) -> (string=w353:string)
                n149 = Delete From Array(array=w363) -> (deleted portion=w371:string, array with subset deleted=w369:string[])  [unwired: 2 in]
                n150 = Array Size(array=w369) -> (size(s)=w367:i32)
                n151 = Initialize Array("\t", w367) -> (w370:string[])
                n152 = Interleave 1D Arrays(w369, w370) -> (w366:string[])
                n153 = Concatenate Strings(w353, w366, w371) -> (w361:string)
              }
              n154 = Build Array (concatenate)("Item", w336) -> (w328:string[])
              n155 = Delete From Array(array=w328) -> (deleted portion=w329:string, array with subset deleted=w331:string[])  [unwired: 2 in]
              n156 = Array Size(array=w331) -> (size(s)=w333:i32)
              n157 = Initialize Array("\t", w333) -> (w330:string[])
              n158 = Interleave 1D Arrays(w331, w330) -> (w334:string[])
              n159 = Concatenate Strings(w334, w329) -> (w319:string)
              n160 = Build Array (concatenate)(w319, w321) -> (w320:string[])
              n161 = Delete From Array(array=w320) -> (deleted portion=w322:string, array with subset deleted=w324:string[])  [unwired: 2 in]
              n162 = Array Size(array=w324) -> (size(s)=w326:i32)
              n163 = Initialize Array("\n", w326) -> (w323:string[])
              n164 = Interleave 1D Arrays(w324, w323) -> (w327:string[])
              n165 = Concatenate Strings(w327, w322) -> (w315:string)
              n166 = Write to Text File(file (use dialog)=w312, text=w315, error in=w313) -> (refnum out=w316:refnum<file>, error out=w317:errorcluster)  [unwired: 1 in, 1 out]
              n167 = case shown="No Error" w317 {
                selector: w317 -> [w348 _]
                tunnel: w316 -> [w347 _]
                tunnel: [w344 w349] -> w314
                tunnel: w313 -> [_ w349]
                frame No Error {
                  n168 = Close File(refnum=w347, error in=w348) -> (path=w345:path, error out=w346:errorcluster)
                  n169 = call "Open in Explore.vi"("error in (no error)"=w346, "path"=w345) -> ("error out"=w344:errorcluster)  [unwired: 9 in]
                }
                frame Error {
                }
              }
            }
            frame Error {
            }
          }
        }
      }
    }
    frame "export_config" {
      n170 = Unbundle By Name(w387) -> ("Properties"=w386:T3[], "Project.ini"=w385:path)
      n171 = for {
        tunnel: w386 -> [w398] mode=indexing
        shift-right: [w396] -> w389
        shift-left: "" -> [w395]
        n172 = Format Into String(format string="%s\n", initial string=w395, w398) -> (resulting string=w396:string)  [unwired: 1 in, 1 out]
      }
      n173 = Open/Create/Replace File(file path (use dialog)=w385, error in=w383, operation (0:open)=T5."replace or create") -> (refnum out=w394:refnum<file>, error out=w393:errorcluster)  [unwired: 3 in, 1 out]
      n174 = Write to Text File(file (use dialog)=w394, text=w389, error in=w393) -> (refnum out=w391:refnum<file>, error out=w392:errorcluster)  [unwired: 1 in, 1 out]
      n175 = Close File(refnum=w391, error in=w392) -> (error out=w384:errorcluster)  [unwired: 1 out]
    }
  }
  "error out" <- w6
  "StateData out" <- w4
